vi "KE622x -- Get Sweep Type.vi"(0 "Resource In":refnum<visa-resource-name>, 1 "Check For SCPI Errors? (T)":bool=TRUE, 11 "error in (no error)":errorcluster) -> (4 "Resource Out (dupl)":refnum<visa-resource-name>, 8 "Sweep Type":T1=enum."Log", 15 "error out":errorcluster)   [LabVIEW 2019, in "Keithley 622x.lvlib"]
doc: "Returns the current active type of sweep, either linear, log, or list sweep."
uses:
  Keithley 622x.lvlib
  Typedefs/KE622x -- Sweep Type.ctl
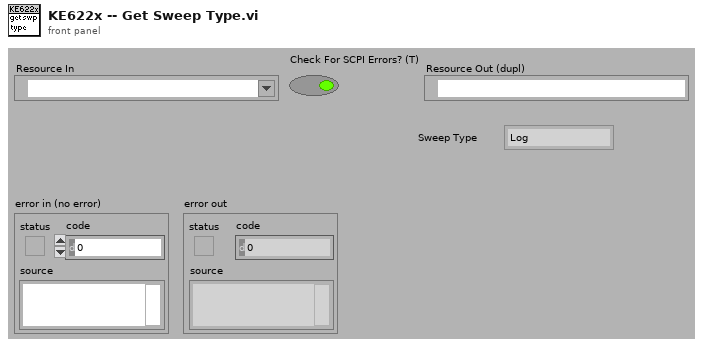
[diagram p1: front panel]
types:
  T1 = typedef "Keithley 622x.lvlib/KE622x -- Sweep Type.ctl" = enum16{"Linear", "Log", "List"}
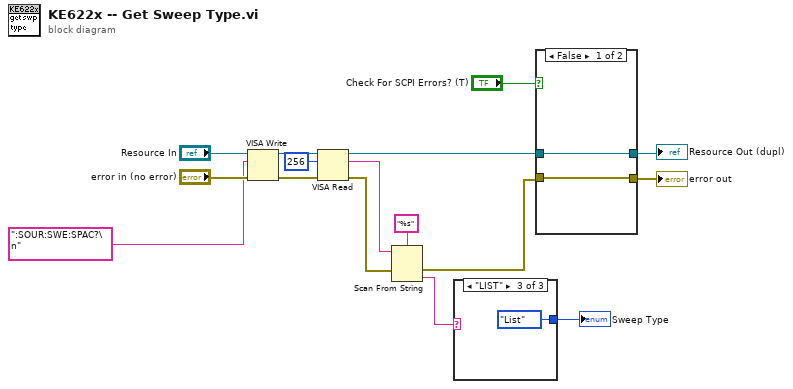
[diagram p0: block diagram]
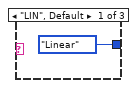
[diagram p2: hidden frame]
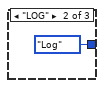
[diagram p3: hidden frame]
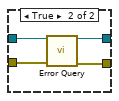
[diagram p4: hidden frame]
diagram:
  n1 = VISA Write(VISA resource name="Resource In", write buffer=":SOUR:SWE:SPAC?\n" ("format string"), error in (no error)="error in (no error)") -> (VISA resource name out=w10:refnum<visa-resource-name>, error out=w9:errorcluster)  [unwired: 1 out]
  n2 = VISA Read(VISA resource name=w10, byte count=u32 256, error in (no error)=w9) -> (VISA resource name out=w3:refnum<visa-resource-name>, read buffer=w5:string, error out=w7:errorcluster)  [unwired: 1 out]
  n3 = Scan From String(format string="%s", input string=w5, error in=w7) -> (error out=w4:errorcluster, output 1=w2:string)  [unwired: 2 in, 2 out]
  n4 = case shown="\"LIST\"" w2 {
    tunnel: [KE622x_--_Sweep_Type."Linear" ("Sweep Type") KE622x_--_Sweep_Type."Log" ("Sweep Type") KE622x_--_Sweep_Type."List" ("Sweep Type")] -> w1
    frame "LIN", Default {
    }
    frame "LOG" {
    }
    frame "LIST" {
    }
  }
  "Sweep Type" <- w1
  n5 = case shown="False" "Check For SCPI Errors? (T)" {
    tunnel: w3 -> [w21 w25]
    tunnel: w4 -> [w20 w24]
    tunnel: [w20 w23] -> w12
    tunnel: [w21 w22] -> w13
    frame False {
    }
    frame True {
      n6 = call "Error Query.vi"("VISA Resource In"=w25, "error in (no error)"=w24) -> ("VISA Resource Out (dupl)"=w22:refnum<visa-resource-name>, "error out"=w23:errorcluster)  [unwired: 10 in, 2 out]
    }
  }
  "Resource Out (dupl)" <- w13
  "error out" <- w12
